vi "Dialog Box.vi"(8 "error in (no error)":errorcluster, 11 "Msg_Error in":refnum<class "ListSelection.lvclass">) -> (0 "error out":errorcluster, 1 "timed out?":bool, 2 "Selection":string, 3 "Msg_Error out":refnum<class "ListSelection.lvclass">)   [LabVIEW 2012, in "ListSelection.lvlib" / "ListSelection.lvclass"]
doc: "This VI contains the code for the dialog box.\nOverride this VI to provide more functionality or to create your own application-specific dialog box."
uses:
  ListSelection.lvclass
  Dialog/Dialog/Dialog.lvclass/Dialog.ctl
  ListSelection.lvclass/ListSelection.ctl
  <vilib>/event_ctls.llb/eventvkey.ctl
  Fading/_Fade In(I32).vi
  Dialog/Dialog/Dialog.lvclass
panel:
  out "String":string
  in  "List":i32[](listbox)
  in  "Accept":bool
  # "Close (or Esc) to Cancel"
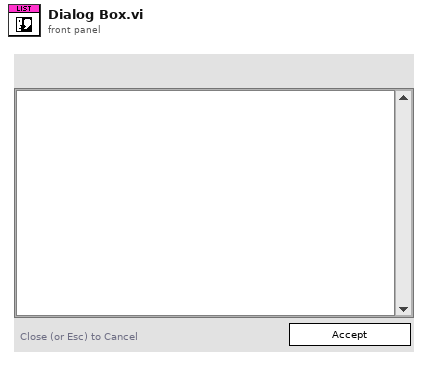
[diagram p1: front panel]
types:
  T1 = typedef "eventvkey.ctl" = enum16{"ASCII", "Enter", "Return", "Shift", "Ctrl", "Alt", "Cmd", "Opt", "Caps", "NumLock", "Clear", "Break", "Up", "Down", "Left", "Right", "Insert", "Delete", "Home", "End", "PageUp", "PageDown", "Escape", "Help", "Pause", "ScrollLock", "F1", "F2", "F3", "F4", "F5", "F6", "F7", "F8", "F9", "F10", "F11", "F12", "F13", "F14", "F15", "F16", "F17", "F18", "F19", "F20", "F21", "F22", "F23", "F24", "Play", "VolumeUp", "VolumeDown", "Mute", "Two Byte Char"}
  T2 = typedef "LVBoundsTypeDef.ctl" = cluster{"Width":u32, "Height":u32}
  T3 = typedef "ListSelection.lvlib/ListSelection.lvclass/Selection Mode.ctl" = enum16{"Zero or one", "One", "Zero or more", "One or more"}
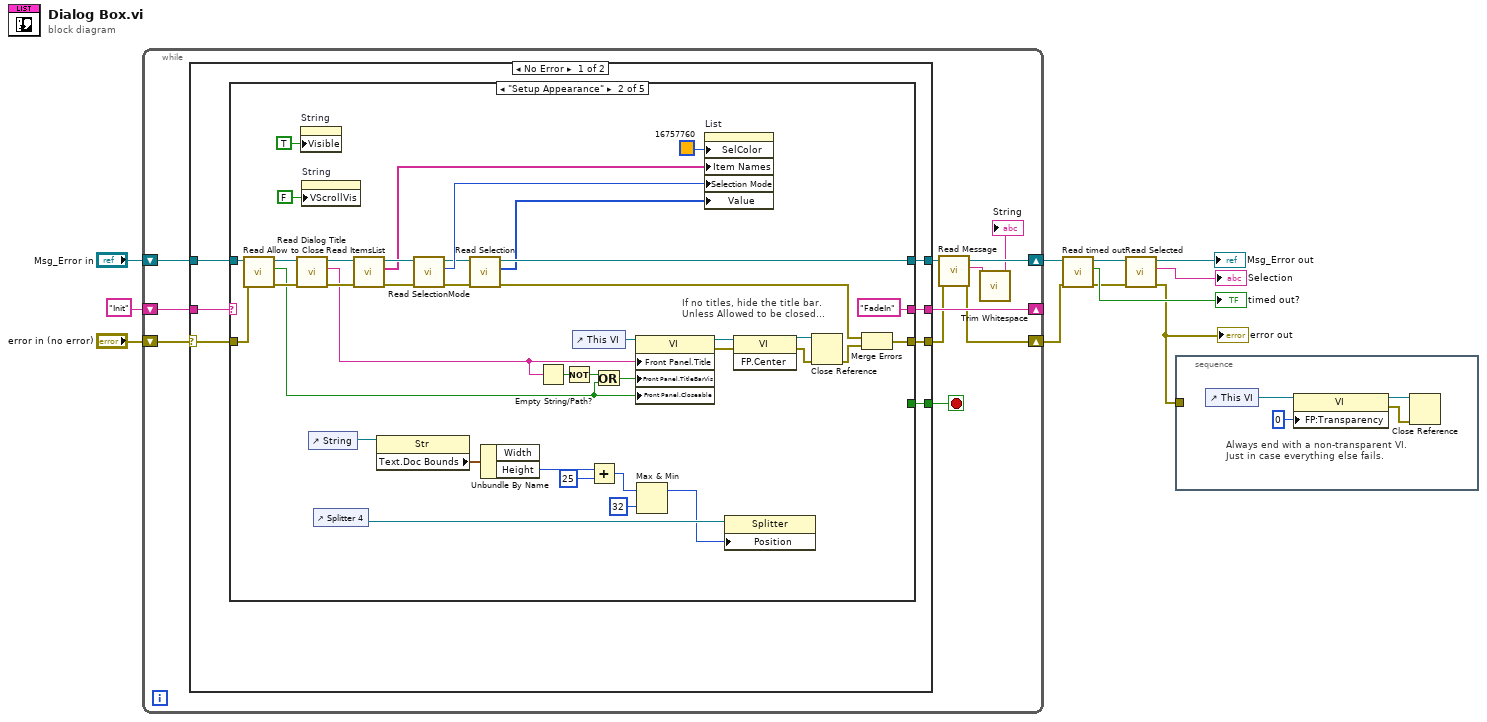
[diagram p0: block diagram]
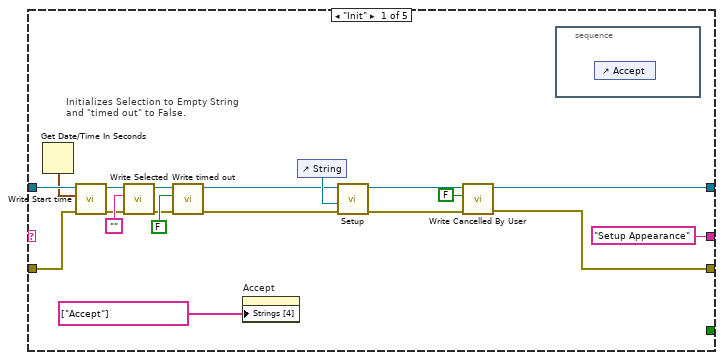
[diagram p2: hidden frame]
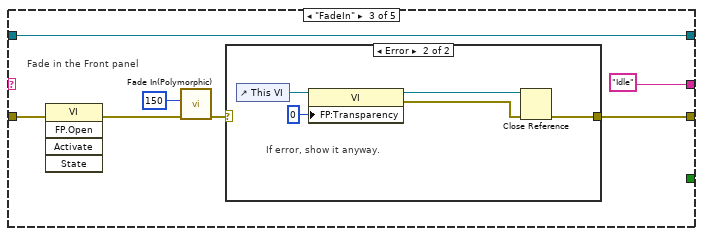
[diagram p3: hidden frame]
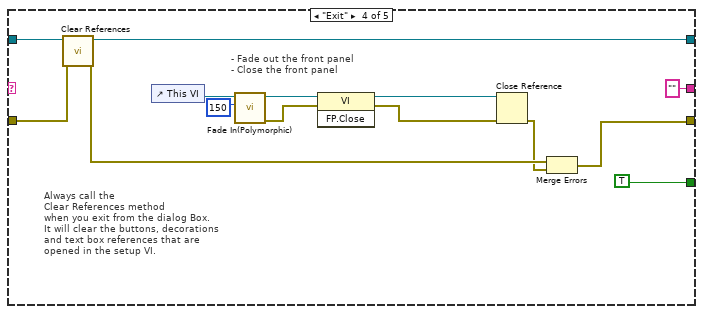
[diagram p5: hidden frame]
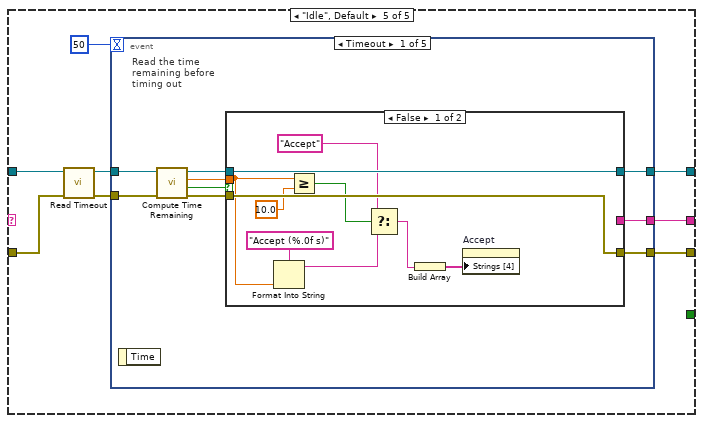
[diagram p6: hidden frame]
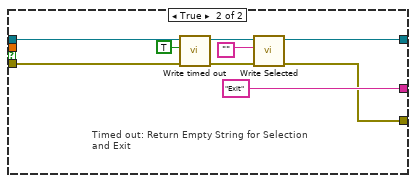
[diagram p7: hidden frame]
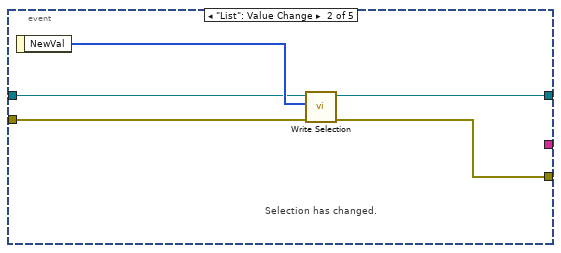
[diagram p8: hidden frame]
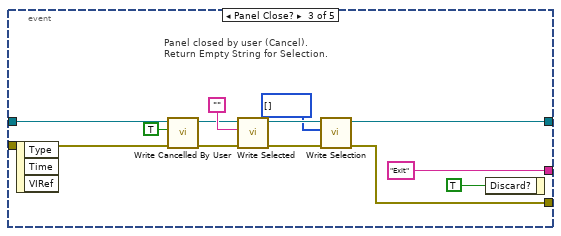
[diagram p9: hidden frame]
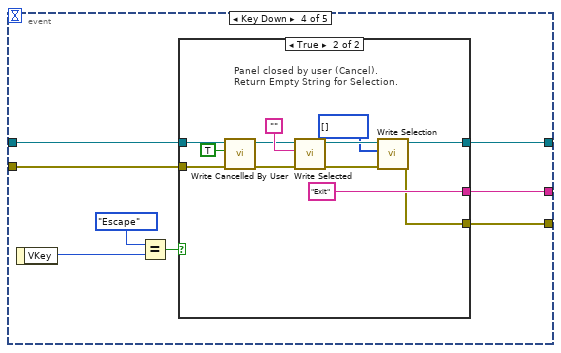
[diagram p10: hidden frame]
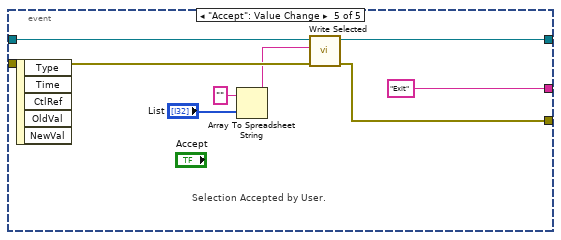
[diagram p12: hidden frame]
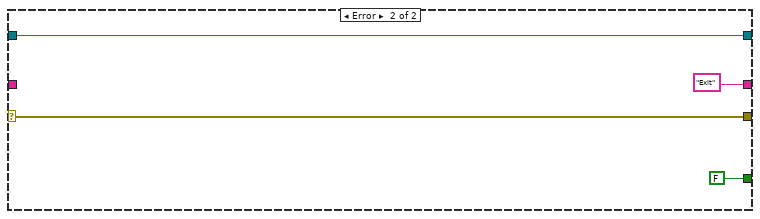
[diagram p13: hidden frame]
diagram:
  n1 = while {
    shift-right: [w20] -> _
    shift-left: "Init" -> [w21]
    shift-right: [w17] -> w5
    shift-left: "Msg_Error in" -> [w22]
    shift-right: [w14] -> w4
    shift-left: "error in (no error)" -> [w18]
    stop <- w19 stop-if-true
    n2 = case shown="No Error" w18 {
      selector: w18 -> [w23 w201]
      tunnel: [w29 w202] -> w16
      tunnel: w22 -> [w28 w202]
      tunnel: [w27 w201] -> w13
      tunnel: w21 -> [w26 _]
      tunnel: [w25 "Exit"] -> w20
      tunnel: [w24 FALSE] -> w19
      frame No Error {
        n3 = case shown="\"Setup Appearance\"" w26 {
          tunnel: [w44 w65 w94 w102 w122] -> w29
          tunnel: w28 -> [w41 w60 w94 w110 w119]
          tunnel: [w43 w61 w88 w101 w121] -> w27
          tunnel: w23 -> [w40 w75 w90 w103 w117]
          tunnel: ["Setup Appearance" "FadeIn" "Idle" "" w120] -> w25
          tunnel: [_ _ _ TRUE _] -> w24
          frame "Init" {
            # "Initializes Selection to Empty String\nand \"timed out\" to False."
            n4 = Get Date/Time In Seconds() -> (seconds since 1Jan1904=w39:timestamp)
            n5 = call "Write Start time.vi"("error in (no error)"=w40, "Start time"=w39, "Dialog in"=w41) -> ("error out"=w33:errorcluster, "Dialog out"=w31:refnum<class "ListSelection.lvclass">)  [unwired: 7 in]
            n6 = call-dynamic "Write Selected.vi"("error in (no error)"=w33, "Selected"="", "Dialog.lvclass in"=w31) -> ("error out"=w34:errorcluster, "Dialog.lvclass out"=w36:refnum<class "ListSelection.lvclass">)  [unwired: 7 out]
            n7 = call-dynamic "Write timed out.vi"("error in (no error)"=w34, "timed out?"=FALSE, "Dialog.lvclass in"=w36) -> ("error out"=w32:errorcluster, "Dialog.lvclass out"=w30:refnum<class "ListSelection.lvclass">)  [unwired: 7 out]
            n8 = property on="Accept" class="Bool"("Strings [4]"=string[] ["Accept"]) -> ()  [unwired: 2 in, 2 out]
            n9 = control-ref of="String"() -> (w47:refnum<vi>)
            n10 = call-dynamic "Setup.vi"("error in (no error)"=w32, "Str Refnum"=w47, "Msg_Error in"=w30) -> ("error out"=w42:errorcluster, "Msg_Error out"=w45:refnum<class "ListSelection.lvclass">)  [unwired: 1 in, 6 out]
            n11 = call "Write Cancelled By User.vi"("error in (no error)"=w42, "cancelled by user?"=FALSE, "Dialog in"=w45) -> ("error out"=w43:errorcluster, "Dialog out"=w44:refnum<class "ListSelection.lvclass">)  [unwired: 7 in]
            n12 = stacked-sequence {
              frame #0 {
                n13 = control-ref of="Accept"() -> ()  [unwired: 1 out]
              }
            }
          }
          frame "Setup Appearance" {
            # "If no titles, hide the title bar.\nUnless Allowed to be closed..."
            n14 = call-dynamic "Read Allow to Close.vi"("error in (no error)"=w75, "Dialog.lvclass in"=w60) -> ("error out"=w79:errorcluster, "Allow to close?"=w76:bool, "Dialog.lvclass out"=w80:refnum<class "ListSelection.lvclass">)  [unwired: 7 out]
            n15 = call-dynamic "Read Dialog Title.vi"("error in (no error)"=w79, "Dialog in"=w80) -> ("error out"=w69:errorcluster, "Dialog Title"=w59:string, "Dialog out"=w64:refnum<class "ListSelection.lvclass">)  [unwired: 7 out]
            n16 = property on="String" class="Str"("Visible"=TRUE) -> ()  [unwired: 2 in, 2 out]
            n17 = property on="String" class="Str"("VScrollVis"=FALSE ("Vertical Scrollbar Visible")) -> ()  [unwired: 2 in, 2 out]
            n18 = control-ref of="String"() -> (w57:refnum<vi>)
            n19 = control-ref of="Splitter 4"() -> (w52:refnum<vi>)
            n20 = call-dynamic "Read ItemsList.vi"("error in (no error)"=w69, "Msg_Error.lvclass in"=w64) -> ("error out"=w68:errorcluster, "Items List"=w71:string[], "Msg_Error.lvclass out"=w72:refnum<class "ListSelection.lvclass">)  [unwired: 7 in]
            n21 = property class="Str"(reference=w57) -> ("Text.Doc Bounds"=w56:T2)  [unwired: 1 in, 2 out]
            n22 = call-dynamic "Read SelectionMode.vi"("error in (no error)"=w68, "Msg_Error.lvclass in"=w72) -> ("error out"=w67:errorcluster, "Selection Mode"=w70:T3, "Msg_Error.lvclass out"=w66:refnum<class "ListSelection.lvclass">)  [unwired: 7 in]
            n23 = call "Read Selection.vi"("error in (no error)"=w67, "ListSelection in"=w66) -> ("error out"=w62:errorcluster, "Selection"=w63:i32[], "ListSelection out"=w65:refnum<class "ListSelection.lvclass">)  [unwired: 7 in]
            n24 = Unbundle By Name(w56) -> ("Height"=w51:u32)  [unwired: 1 out]
            n25 = Empty String/Path?(string/path=w59) -> (empty?=w85:bool)
            n26 = Not(x=w85) -> (.not. x?=w78:bool)
            n27 = control-ref of="This VI"() -> (w86:refnum<vi>)
            n28 = Add(x=w51, y=u32 25) -> (x+y=w53:u32)
            n29 = Or(x=w78, y=w76) -> (x .or. y?=w77:bool)
            n30 = property class="VI"(reference=w86, "Front Panel.Title"=w59, "Front Panel.TitleBarVis"=w77, "Front Panel.Closeable"=w76) -> (reference out=w84:refnum<vi>, error out=w83:errorcluster)  [unwired: 1 in]
            n31 = Max & Min(x=w53, y=u32 32) -> (max(x,y)=w50:u32)  [unwired: 1 out]
            n32 = property on="List" class="LstBox (strict)"("SelColor"=u32 16757760, "Item Names"=w71, "Selection Mode"=w70, "Value"=w63) -> ()  [unwired: 2 in, 2 out]
            n33 = property class="Splitter"(reference=w52, "Position"=w50) -> ()  [unwired: 1 in, 2 out]
            n34 = invoke class="VI" method="FP.Center"(reference=w84, error in=w83) -> (reference out=w82:refnum<vi>, error out=w81:errorcluster)  [unwired: 1 in, 1 out]
            n35 = Close Reference(reference=w82, error in (no error)=w81) -> (error out=w58:errorcluster)
            n36 = Merge Errors(w62, w58) -> (w61:errorcluster)
          }
          frame "FadeIn" {
            # "Fade in the Front panel"
            n37 = invoke class="VI" method="FP.Open"(error in=w90) -> (error out=w89:errorcluster)  [unwired: 4 in, 4 out]
            n38 = call-poly "Fade In(Polymorphic).vi"("error in"=w89, "Fade time (ms)"=150) -> ("error out"=w91:errorcluster)  [unwired: 2 in, 7 out]
            n39 = case shown="Error" w91 {
              selector: w91 -> [w95 _]
              tunnel: [w95 w96] -> w88
              frame No Error {
              }
              frame Error {
                # "If error, show it anyway."
                n40 = control-ref of="This VI"() -> (w98:refnum<vi>)
                n41 = property class="VI"(reference=w98, "FP:Transparency"=u8 0 ("Front Panel Window:Transparency")) -> (reference out=w99:refnum<vi>, error out=w100:errorcluster)  [unwired: 1 in]
                n42 = Close Reference(reference=w99, error in (no error)=w100) -> (error out=w96:errorcluster)
              }
            }
          }
          frame "Exit" {
            # "Always call the\nClear References method\nwhen you exit from the dialog Box.\nIt will clear the buttons, decorations\nand text box references that are \nopened in the setup VI."
            # "- Fade out the front panel\n- Close the front panel"
            n43 = call-dynamic "Clear References.vi"("error in (no error)"=w103, "Dialog in"=w110) -> ("error out"=w105:errorcluster, "Dialog out"=w102:refnum<class "ListSelection.lvclass">)  [unwired: 8 out]
            n44 = control-ref of="This VI"() -> (w111:refnum<vi>)
            n45 = call-poly "Fade In(Polymorphic).vi"("Fade time (ms)"=150, "VI Reference (calling VI)"=w111) -> ("error out"=w109:errorcluster, "dup VI Reference"=w108:refnum<vi>)  [unwired: 2 in, 6 out]
            n46 = invoke class="VI" method="FP.Close"(reference=w108, error in=w109) -> (reference out=w106:refnum<vi>, error out=w107:errorcluster)  [unwired: 1 in, 1 out]
            n47 = Close Reference(reference=w106, error in (no error)=w107) -> (error out=w104:errorcluster)
            n48 = Merge Errors(w105, w104) -> (w101:errorcluster)
          }
          frame "Idle", Default {
            n49 = call-dynamic "Read Timeout.vi"("error in (no error)"=w117, "Dialog.lvclass in"=w119) -> ("error out"=w116:errorcluster, "Dialog.lvclass out"=w118:refnum<class "ListSelection.lvclass">)  [unwired: 8 out]
            n50 = event shown="[0] Timeout" {
              selector: _ -> [_ _ _ _ _]
              dyn-events: _ -> [_ _ _ _ _]
              timeout: 50 -> [_ _ _ _ _]
              tunnel: [w129 w151 w164 w175 w196] -> w122
              tunnel: w118 -> [w126 w154 w160 w173 w197]
              tunnel: [w130 w152 w162 w174 w194] -> w121
              tunnel: w116 -> [w128 w153 w158 w172 w195]
              tunnel: [w131 _ "Exit" w176 "Exit"] -> w120
              event Timeout {
                # "Read the time remaining before timing out"
                n51 = event-data() -> ()  [unwired: 2 out]
                n52 = call "Compute Time Remaining.vi"("error in (no error)"=w128, "Dialog in"=w126) -> ("error out"=w127:errorcluster, "Elapsed"=w124:bool, "Time remaining (s)"=w123:dbl, "Dialog out"=w125:refnum<class "ListSelection.lvclass">)  [unwired: 6 in]
                n53 = case shown="False" w124 {
                  tunnel: [_ "Exit"] -> w131
                  tunnel: [w140 w146] -> w130
                  tunnel: [w141 w145] -> w129
                  tunnel: w127 -> [w140 w143]
                  tunnel: w125 -> [w141 w142]
                  tunnel: w123 -> [w137 _]
                  frame False {
                    n54 = Format Into String(format string="Accept (%.0f s)", w137) -> (resulting string=w135:string)  [unwired: 2 in, 1 out]
                    n55 = Greater Or Equal?(x=w137, y=10.0) -> (x >= y?=w134:bool)
                    n56 = Select(t="Accept", s=w134, f=w135) -> (s? t:f=w133:string)
                    n57 = Build Array(w133) -> (w132:string[])
                    n58 = property on="Accept" class="Bool"("Strings [4]"=w132) -> ()  [unwired: 2 in, 2 out]
                  }
                  frame True {
                    # "Timed out: Return Empty String for Selection\nand Exit"
                    n59 = call-dynamic "Write timed out.vi"("error in (no error)"=w143, "timed out?"=TRUE, "Dialog.lvclass in"=w142) -> ("error out"=w147:errorcluster, "Dialog.lvclass out"=w148:refnum<class "ListSelection.lvclass">)  [unwired: 7 out]
                    n60 = call-dynamic "Write Selected.vi"("error in (no error)"=w147, "Selected"="", "Dialog.lvclass in"=w148) -> ("error out"=w146:errorcluster, "Dialog.lvclass out"=w145:refnum<class "ListSelection.lvclass">)  [unwired: 7 out]
                  }
                }
              }
              event "List": Value Change {
                # "Selection has changed."
                n61 = event-data() -> ("NewVal"=w155:i32[])  [unwired: 1 out]
                n62 = call "Write Selection.vi"("error in (no error)"=w153, "Selection"=w155, "ListSelection in"=w154) -> ("error out"=w152:errorcluster, "ListSelection out"=w151:refnum<class "ListSelection.lvclass">)  [unwired: 7 in]
              }
              event Panel Close? {
                # "Panel closed by user (Cancel).\nReturn Empty String for Selection."
                n63 = event-data() -> ()  [unwired: 4 out]
                n64 = call "Write Cancelled By User.vi"("error in (no error)"=w158, "cancelled by user?"=TRUE, "Dialog in"=w160) -> ("error out"=w157:errorcluster, "Dialog out"=w159:refnum<class "ListSelection.lvclass">)  [unwired: 7 in]
                n65 = call-dynamic "Write Selected.vi"("error in (no error)"=w157, "Selected"="", "Dialog.lvclass in"=w159) -> ("error out"=w163:errorcluster, "Dialog.lvclass out"=w165:refnum<class "ListSelection.lvclass">)  [unwired: 7 out]
                n66 = call "Write Selection.vi"("error in (no error)"=w163, "Selection"=i32[] [], "ListSelection in"=w165) -> ("error out"=w162:errorcluster, "ListSelection out"=w164:refnum<class "ListSelection.lvclass">)  [unwired: 7 in]
                n67 = event-data("Discard?"=TRUE) -> ()  [unwired: 1 in, 1 out]
              }
              event Key Down {
                n68 = event-data() -> ("VKey"=w171:T1)  [unwired: 1 out]
                n69 = Equal?(x=eventvkey."Escape" ("VKey"), y=w171) -> (x = y?=w169:bool)
                n70 = case shown="True" w169 {
                  tunnel: [_ "Exit"] -> w176
                  tunnel: [w178 w187] -> w175
                  tunnel: [w177 w185] -> w174
                  tunnel: w173 -> [w178 w183]
                  tunnel: w172 -> [w177 w181]
                  frame False {
                  }
                  frame True {
                    # "Panel closed by user (Cancel).\nReturn Empty String for Selection."
                    n71 = call "Write Cancelled By User.vi"("error in (no error)"=w181, "cancelled by user?"=TRUE, "Dialog in"=w183) -> ("error out"=w180:errorcluster, "Dialog out"=w182:refnum<class "ListSelection.lvclass">)  [unwired: 7 in]
                    n72 = call-dynamic "Write Selected.vi"("error in (no error)"=w180, "Selected"="", "Dialog.lvclass in"=w182) -> ("error out"=w186:errorcluster, "Dialog.lvclass out"=w188:refnum<class "ListSelection.lvclass">)  [unwired: 7 out]
                    n73 = call "Write Selection.vi"("error in (no error)"=w186, "Selection"=i32[] [], "ListSelection in"=w188) -> ("error out"=w185:errorcluster, "ListSelection out"=w187:refnum<class "ListSelection.lvclass">)  [unwired: 7 in]
                  }
                }
              }
              event "Accept": Value Change {
                # "Selection Accepted by User."
                n74 = event-data() -> ()  [unwired: 6 out]
                n75 = Array To Spreadsheet String(array="List", 3:"" ("format string")) -> (spreadsheet string=w191:string)  [unwired: 1 in]
                n76 = call-dynamic "Write Selected.vi"("error in (no error)"=w195, "Selected"=w191, "Dialog.lvclass in"=w197) -> ("error out"=w194:errorcluster, "Dialog.lvclass out"=w196:refnum<class "ListSelection.lvclass">)  [unwired: 7 out]
              }
            }
          }
        }
      }
      frame Error {
      }
    }
    n77 = call-dynamic "Read Message.vi"("error in (no error)"=w13, "Dialog in"=w16) -> ("error out"=w14:errorcluster, "Message"=w15:string, "Dialog out"=w17:refnum<class "ListSelection.lvclass">)  [unwired: 7 in]
    n78 = call <vilib>:"Trim Whitespace.vi"("string"=w15) -> ("trimmed string"=→"String":string)  [unwired: 1 in]
  }
  n79 = call-dynamic "Read timed out.vi"("error in (no error)"=w4, "Dialog.lvclass in"=w5) -> ("error out"=w2:errorcluster, "timed out?"=→"timed out?":bool, "Dialog.lvclass out"=w3:refnum<class "ListSelection.lvclass">)  [unwired: 7 out]
  n80 = call-dynamic "Read Selected.vi"("error in (no error)"=w2, "Dialog.lvclass in"=w3) -> ("error out"=w1:errorcluster, "Selected"=→"Selection":string, "Dialog.lvclass out"=→"Msg_Error out":refnum<class "ListSelection.lvclass">)  [unwired: 7 out]
  "error out" <- w1
  n81 = stacked-sequence {
    tunnel: w1 -> [_]
    frame #0 {
      # "Always end with a non-transparent VI.\nJust in case everything else fails."
      n82 = control-ref of="This VI"() -> (w205:refnum<vi>)
      n83 = property class="VI"(reference=w205, "FP:Transparency"=u8 0 ("Front Panel Window:Transparency")) -> (reference out=w204:refnum<vi>, error out=w203:errorcluster)  [unwired: 1 in]
      n84 = Close Reference(reference=w204, error in (no error)=w203) -> ()  [unwired: 1 out]
    }
  }
